vi "Autonomous Independent.vi"() -> ()   [LabVIEW 2018]
doc: "This VI is called when autonomous begins, and will automatically be terminated when autonomous ends. You can carry out timed or sensor driven robot movement independently without needing to return to the caller."
uses:
  State Machines/autos.ctl
  <vilib>/Rock Robotics/WPI/DriverStation/WPI_DriverStationRobotMode2.ctl
  Robot Global Data.vi
  <vilib>/Rock Robotics/Network Tables/NT Read Number.vi
  <vilib>/Rock Robotics/WPI/Utilities/WPI_GetSetVariantRefNum.vi
  Support Code/Valkyrie1Buttons.vi
panel:
  in  "Range":cluster{"output high":dbl, "output low":dbl}={"output high"=0.7, "output low"=-0.6}
  in  "Gains":T1={"proportional gain (Kc)"=0.03, "integral time (Ti, min)"=0.01, "derivative time (Td, min)"=0.0}
  in  "Time to stop R":i32=1000
  in  "Distance fwd r":dbl=700.0 format="%#_13g"
  in  "Time to Wait r":dbl=100.0
  in  "Distance fwd 1":dbl=200.0 format="%#_13g"
  in  "Time to stop":i32=1000
  out "Finished?":bool
  in  "Time to Wait":dbl=100.0
  # "Ganhos PID"
  # "Cargo Ship"
  # "Rocket"
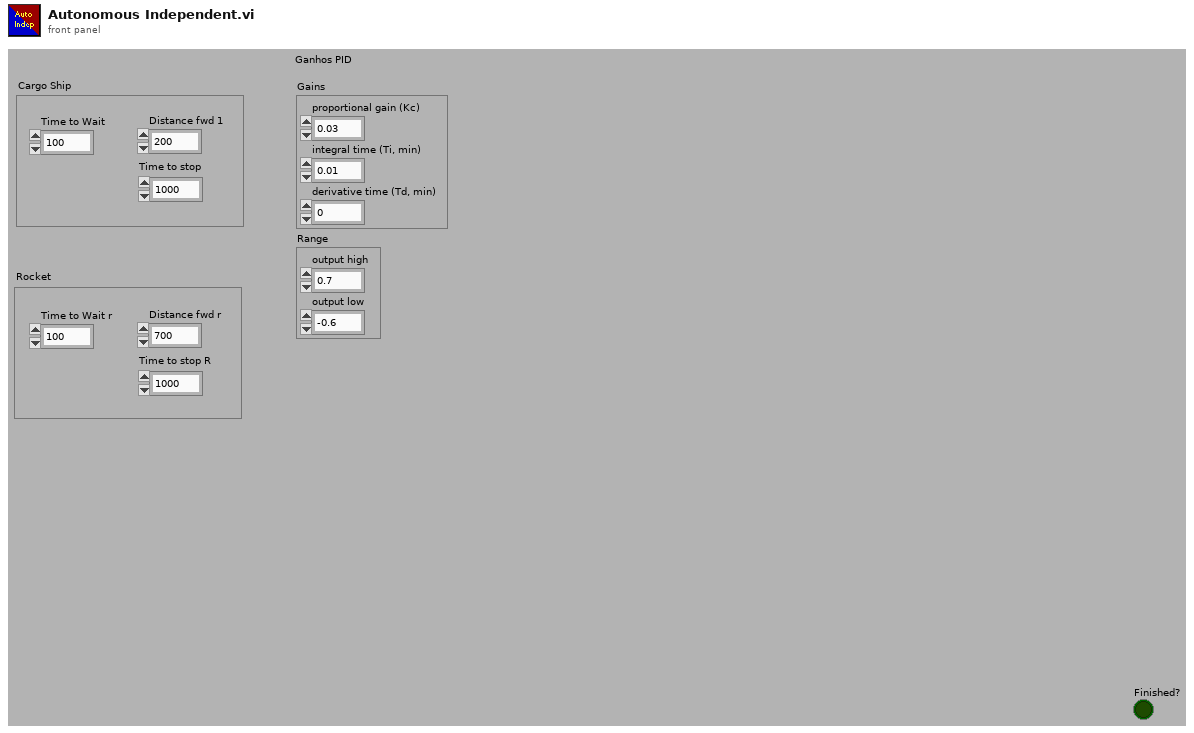
[diagram p1: front panel]
types:
  T1 = cluster{"proportional gain (Kc)":dbl, "integral time (Ti, min)":dbl, "derivative time (Td, min)":dbl}
  T2 = typedef "autos.ctl" = enum16{"Airship", " Rocket", "Anda"}
  T3 = enum16{"ZerandoSensor", "Frente1", "DriverAlinha", "Pontua", "Fim"}
  T4 = typedef "WPI_DriverStationRobotMode2.ctl" = enum16{"Autonomous Disabled", "Autonomous Enabled", "Teleop Disabled", "Teleop Enabled", "Disconnected", "Finish", "Test Disabled", "Test Enabled", "Emergency Stopped"}
  T5 = typedef "WPI_JoystickDevRef.ctl" = cluster{"Device":T6}
  T6 = typedef "WPI_JoystickDeviceEnum.ctl" = enum16{"USB 0", "USB 1", "USB 2", "USB 3", "USB 4", "USB 5"}
  T7 = typedef "D-Pad.ctl" = cluster{"Top":bool, "Bottom":bool, "None":bool, "Right":bool, "Left":bool}
  T8 = typedef "Button Cluster.ctl" = cluster{"Buttons[0]":bool, "Buttons[1]":bool, "Buttons[2]":bool, "Buttons[3]":bool, "Buttons[4]":bool, "Buttons[5]":bool, "Buttons[6]":bool, "Buttons[7]":bool, "Buttons[8]":bool, "Buttons[9]":bool}
  T9 = typedef "Axes Cluster.ctl" = cluster{"Axes[0]":dbl, "Axes[1]":dbl, "Axes[2]":dbl, "Axes[3]":dbl, "Axes[4]":dbl, "Axes[5]":dbl, "Axes[6]":dbl, "Axes[7]":dbl, "Axes[8]":dbl}
  T10 = typedef "WPI_EncoderDevRef.ctl" = cluster{"DevStatus":errorcluster, "EncoderIndex":T11, "CounterIndex":T12, "DistancePerCount":dbl, "Decoding Type":T13}
  T11 = typedef "FPGA_EncoderIdx.ctl" = enum8{"Enc 0", "Enc 1", "Enc 2", "Enc 3", "Enc 4", "Enc 5", "Enc 6", "Enc 7", "Invalid"}
  T12 = typedef "FPGA_CounterCtrSystemIndex.ctl" = enum8{"Ctr 0", "Ctr 1", "Ctr 2", "Ctr 3", "Ctr 4", "Ctr 5", "Ctr 6", "Ctr 7", "Invalid"}
  T13 = typedef "WPI_EncoderType.ctl" = enum16{"1x", "2x", "4x"}
  T14 = cluster{"Yaw":dbl, "Roll":dbl, "Pitch":dbl, "Heading":dbl, "Fused Heading":dbl}
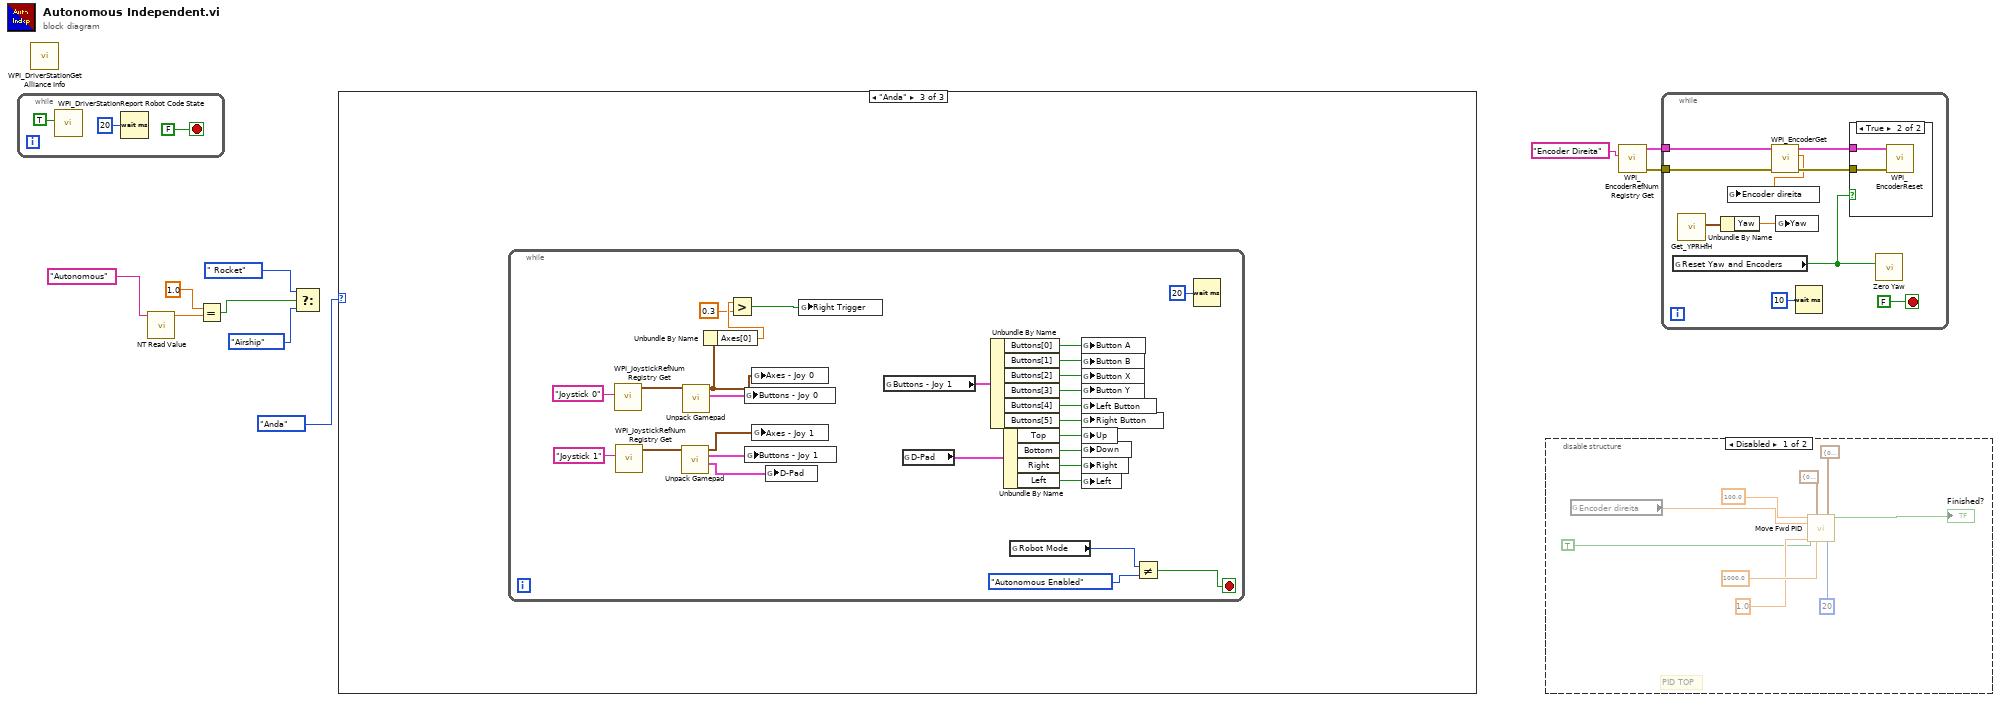
[diagram p0: block diagram]
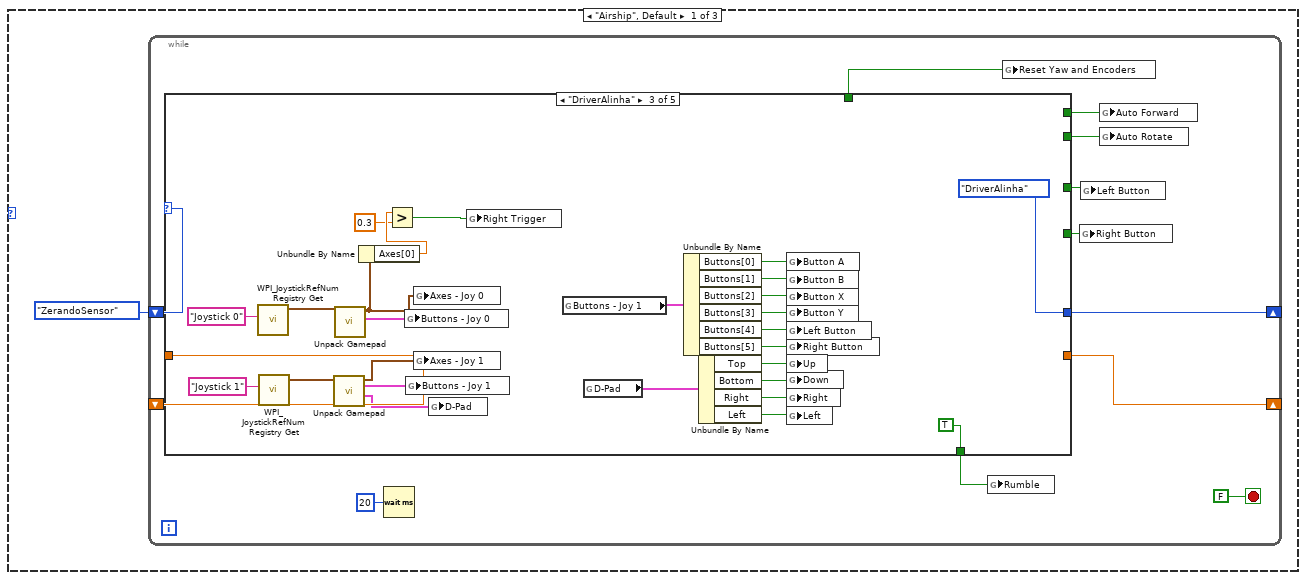
[diagram p4: hidden frame]
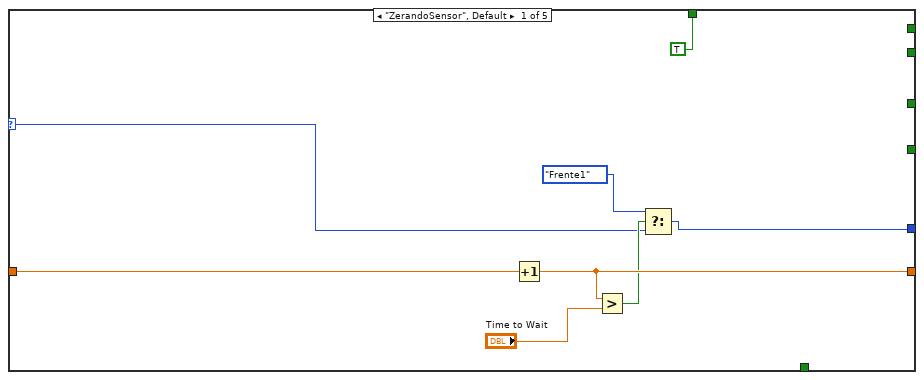
[diagram p5: hidden frame]
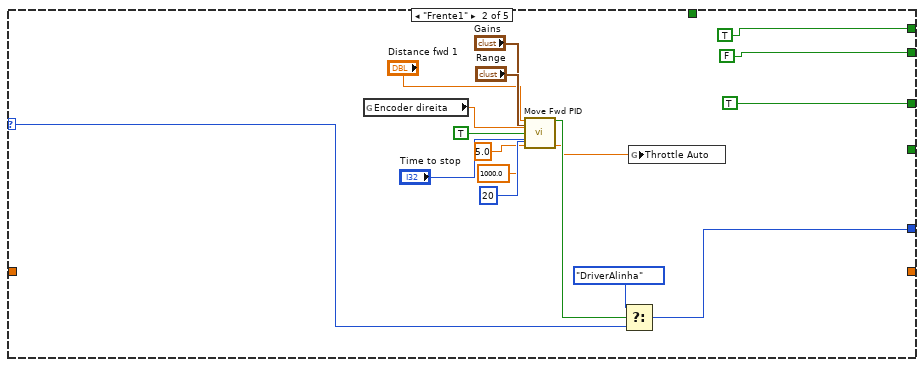
[diagram p6: hidden frame]
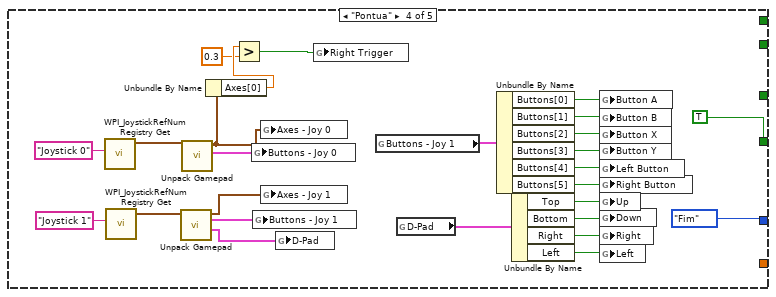
[diagram p7: hidden frame]
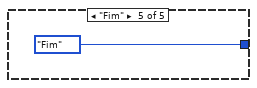
[diagram p8: hidden frame]
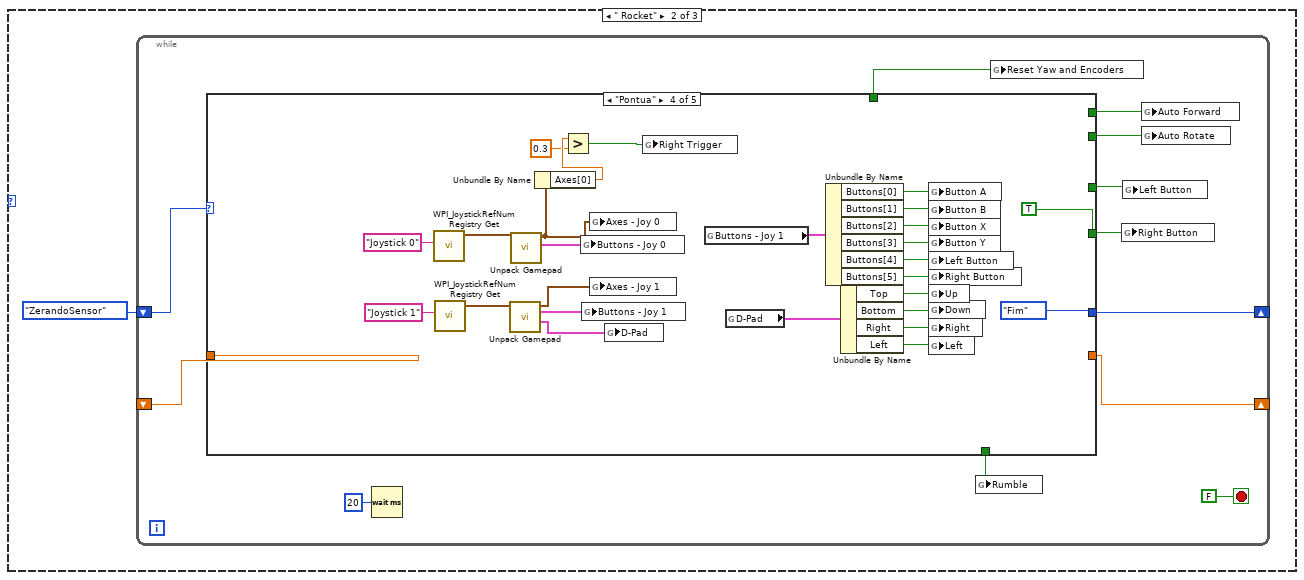
[diagram p9: hidden frame]
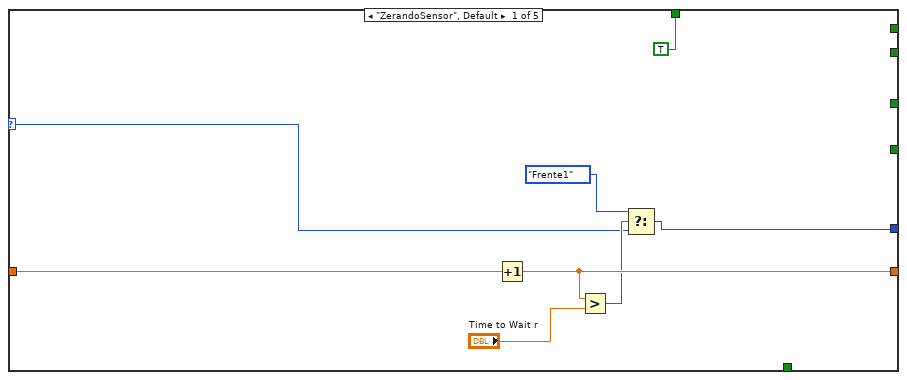
[diagram p10: hidden frame]
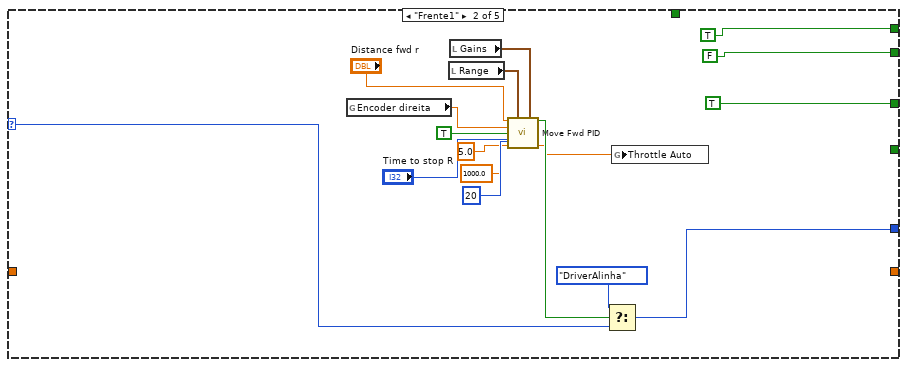
[diagram p11: hidden frame]
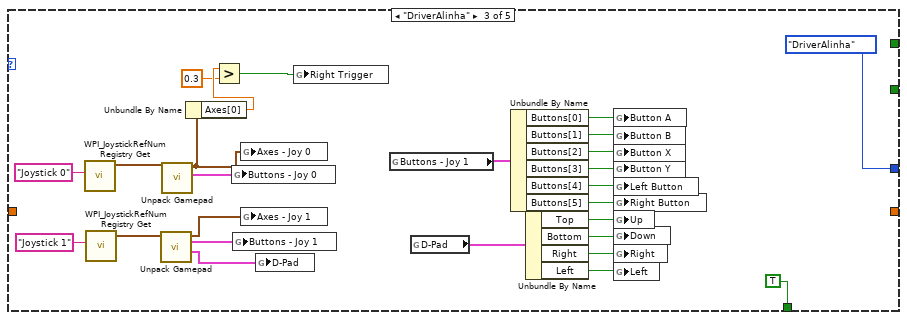
[diagram p12: hidden frame]
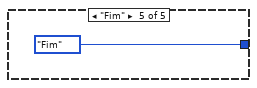
[diagram p13: hidden frame]
diagram:
  n1 = while {
    stop <- FALSE stop-if-true
    n2 = call <vilib>:"WPI_DriverStationReport Robot Code State.vi"("Autonomous"=TRUE) -> ()  [unwired: 10 in, 1 out]
    n3 = Wait (ms)(milliseconds to wait=u32 20) -> ()  [unwired: 1 out]
  }
  n4 = call <vilib>:"WPI_DriverStationGet Alliance Info.vi"() -> ()  [unwired: 12 out]
  n5 = call-poly <vilib>:"NT Read Value.vi"("Name"="Autonomous") -> ("Numeric"=w6:dbl)  [unwired: 9 in, 1 out]
  n6 = Equal?(x=1.0, y=w6) -> (x = y?=w2:bool)
  n7 = Select(t=autos." Rocket", s=w2, f=autos."Airship") -> ()  [unwired: 1 out]
  n8 = case shown="\"Anda\"" autos."Anda" {
    frame "Airship", Default {
      n9 = while {
        shift-right: [w23] -> _
        shift-left: _ -> [w24]
        shift-right: [w20] -> _
        shift-left: T3."ZerandoSensor" -> [w21]
        stop <- FALSE stop-if-true
        n10 = case shown="\"DriverAlinha\"" w21 {
          selector: w21 -> [w28 w50 _ _ _]
          tunnel: [TRUE _ _ _ _] -> w25
          tunnel: w24 -> [w33 _ _ _ _]
          tunnel: [w32 _ _ _ _] -> w23
          tunnel: [w30 w51 T3."DriverAlinha" ("t") T3."Fim" ("t") T3."Fim" ("t")] -> w20
          tunnel: [_ TRUE _ _ _] -> w19
          tunnel: [_ FALSE _ _ _] -> w18
          tunnel: [_ TRUE _ _ _] -> w17
          tunnel: [_ _ _ TRUE _] -> w16
          tunnel: [_ _ TRUE _ _] -> w15
          frame "ZerandoSensor", Default {
            n11 = Increment(x=w33) -> (x+1=w32:dbl)
            n12 = Greater?(x=w32, y="Time to Wait") -> (0:w29:bool)
            n13 = Select(t=T3."Frente1", s=w29, f=w28) -> (s? t:f=w30:T3)
          }
          frame "Frente1" {
            n14 = global read "Robot Global Data.vi" "Encoder direita"() -> (w48:dbl)
            n15 = call "Move Fwd PID.vi"("Distance"="Distance fwd 1", "Range"="Range", "Gains"="Gains", "Encoder Count"=w48, "Reset Rate"=TRUE, "Time to stop"="Time to stop", "Precision"=5.0, "Soft start"=1000.0, "Loop Timer"=20) -> ("Finished?"=w39:bool, "Output"=w35:dbl)  [unwired: 5 in]
            n16 = Select(t=T3."DriverAlinha", s=w39, f=w50) -> (s? t:f=w51:T3)
            n17 = global write "Robot Global Data.vi" "Throttle Auto"(w35) -> ()
          }
          frame "DriverAlinha" {
            n18 = call <vilib>:"WPI_JoystickRefNum Registry Get.vi"("refnum name"="Joystick 0") -> ("JoystickDevRef"=w74:T5)  [unwired: 1 in, 9 out]
            n19 = call <vilib>:"WPI_JoystickRefNum Registry Get.vi"("refnum name"="Joystick 1") -> ("JoystickDevRef"=w73:T5)  [unwired: 1 in, 9 out]
            n20 = call "Unpack Gamepad.vi"("JoystickDevRef"=w73) -> ("D-Pad"=w71:T7, "Button Cluster"=w70:T8, "Axes"=w69:T9)  [unwired: 8 in]
            n21 = call "Unpack Gamepad.vi"("JoystickDevRef"=w74) -> ("Button Cluster"=w72:T8, "Axes"=w68:T9)  [unwired: 8 in, 1 out]
            n22 = Unbundle By Name(w68) -> ("Axes[0]"=w67:dbl)
            n23 = Greater?(x=w67, y=0.3) -> (0:w65:bool)
            n24 = global write "Robot Global Data.vi" "Buttons - Joy 0"(w72) -> ()
            n25 = global write "Robot Global Data.vi" "Buttons - Joy 1"(w70) -> ()
            n26 = global write "Robot Global Data.vi" "Axes - Joy 0"(w68) -> ()
            n27 = global write "Robot Global Data.vi" "Axes - Joy 1"(w69) -> ()
            n28 = global write "Robot Global Data.vi" "D-Pad"(w71) -> ()
            n29 = global write "Valkyrie1Buttons.vi" "Right Trigger"(w65) -> ()
            n30 = global read "Robot Global Data.vi" "Buttons - Joy 1"() -> (w64:T8)
            n31 = global read "Robot Global Data.vi" "D-Pad"() -> (w63:T7)
            n32 = Unbundle By Name(w64) -> ("Buttons[0]"=w62:bool, "Buttons[1]"=w61:bool, "Buttons[2]"=w60:bool, "Buttons[3]"=w59:bool, "Buttons[4]"=w53:bool, "Buttons[5]"=w54:bool)
            n33 = Unbundle By Name(w63) -> ("Top"=w55:bool, "Bottom"=w56:bool, "Right"=w57:bool, "Left"=w58:bool)
            n34 = global write "Valkyrie1Buttons.vi" "Button A"(w62) -> ()
            n35 = global write "Valkyrie1Buttons.vi" "Button B"(w61) -> ()
            n36 = global write "Valkyrie1Buttons.vi" "Button X"(w60) -> ()
            n37 = global write "Valkyrie1Buttons.vi" "Button Y"(w59) -> ()
            n38 = global write "Valkyrie1Buttons.vi" "Left Button"(w53) -> ()
            n39 = global write "Valkyrie1Buttons.vi" "Right Button"(w54) -> ()
            n40 = global write "Valkyrie1Buttons.vi" "Up"(w55) -> ()
            n41 = global write "Valkyrie1Buttons.vi" "Down"(w56) -> ()
            n42 = global write "Valkyrie1Buttons.vi" "Right"(w57) -> ()
            n43 = global write "Valkyrie1Buttons.vi" "Left"(w58) -> ()
          }
          frame "Pontua" {
            n44 = call <vilib>:"WPI_JoystickRefNum Registry Get.vi"("refnum name"="Joystick 0") -> ("JoystickDevRef"=w99:T5)  [unwired: 1 in, 9 out]
            n45 = call <vilib>:"WPI_JoystickRefNum Registry Get.vi"("refnum name"="Joystick 1") -> ("JoystickDevRef"=w98:T5)  [unwired: 1 in, 9 out]
            n46 = call "Unpack Gamepad.vi"("JoystickDevRef"=w98) -> ("D-Pad"=w96:T7, "Button Cluster"=w95:T8, "Axes"=w94:T9)  [unwired: 8 in]
            n47 = call "Unpack Gamepad.vi"("JoystickDevRef"=w99) -> ("Button Cluster"=w97:T8, "Axes"=w81:T9)  [unwired: 8 in, 1 out]
            n48 = Unbundle By Name(w81) -> ("Axes[0]"=w80:dbl)
            n49 = Greater?(x=w80, y=0.3) -> (0:w78:bool)
            n50 = global write "Robot Global Data.vi" "Buttons - Joy 0"(w97) -> ()
            n51 = global write "Robot Global Data.vi" "Buttons - Joy 1"(w95) -> ()
            n52 = global write "Robot Global Data.vi" "Axes - Joy 0"(w81) -> ()
            n53 = global write "Robot Global Data.vi" "Axes - Joy 1"(w94) -> ()
            n54 = global write "Robot Global Data.vi" "D-Pad"(w96) -> ()
            n55 = global write "Valkyrie1Buttons.vi" "Right Trigger"(w78) -> ()
            n56 = global read "Robot Global Data.vi" "Buttons - Joy 1"() -> (w93:T8)
            n57 = global read "Robot Global Data.vi" "D-Pad"() -> (w92:T7)
            n58 = Unbundle By Name(w93) -> ("Buttons[0]"=w91:bool, "Buttons[1]"=w90:bool, "Buttons[2]"=w89:bool, "Buttons[3]"=w88:bool, "Buttons[4]"=w82:bool, "Buttons[5]"=w83:bool)
            n59 = Unbundle By Name(w92) -> ("Top"=w84:bool, "Bottom"=w85:bool, "Right"=w86:bool, "Left"=w87:bool)
            n60 = global write "Valkyrie1Buttons.vi" "Button A"(w91) -> ()
            n61 = global write "Valkyrie1Buttons.vi" "Button B"(w90) -> ()
            n62 = global write "Valkyrie1Buttons.vi" "Button X"(w89) -> ()
            n63 = global write "Valkyrie1Buttons.vi" "Button Y"(w88) -> ()
            n64 = global write "Valkyrie1Buttons.vi" "Left Button"(w82) -> ()
            n65 = global write "Valkyrie1Buttons.vi" "Right Button"(w83) -> ()
            n66 = global write "Valkyrie1Buttons.vi" "Up"(w84) -> ()
            n67 = global write "Valkyrie1Buttons.vi" "Down"(w85) -> ()
            n68 = global write "Valkyrie1Buttons.vi" "Right"(w86) -> ()
            n69 = global write "Valkyrie1Buttons.vi" "Left"(w87) -> ()
          }
          frame "Fim" {
          }
        }
        n70 = Wait (ms)(milliseconds to wait=u32 20) -> ()  [unwired: 1 out]
        n71 = global write "Robot Global Data.vi" "Rumble"(w15) -> ()
        n72 = global write "Robot Global Data.vi" "Reset Yaw and Encoders"(w25) -> ()
        n73 = global write "Valkyrie1Buttons.vi" "Right Button"(w16) -> ()
        n74 = global write "Valkyrie1Buttons.vi" "Left Button"(w17) -> ()
        n75 = global write "Robot Global Data.vi" "Auto Forward"(w19) -> ()
        n76 = global write "Robot Global Data.vi" "Auto Rotate"(w18) -> ()
      }
    }
    frame " Rocket" {
      n77 = while {
        shift-right: [w114] -> _
        shift-left: _ -> [w115]
        shift-right: [w111] -> _
        shift-left: T3."ZerandoSensor" -> [w112]
        stop <- FALSE stop-if-true
        n78 = case shown="\"Pontua\"" w112 {
          selector: w112 -> [w119 w141 _ _ _]
          tunnel: [TRUE _ _ _ _] -> w116
          tunnel: w115 -> [w124 _ _ _ _]
          tunnel: [w123 _ _ _ _] -> w114
          tunnel: [w121 w142 T3."DriverAlinha" ("t") T3."Fim" ("t") T3."Fim" ("t")] -> w111
          tunnel: [_ TRUE _ _ _] -> w110
          tunnel: [_ FALSE _ _ _] -> w109
          tunnel: [_ TRUE _ _ _] -> w108
          tunnel: [_ _ _ TRUE _] -> w107
          tunnel: [_ _ TRUE _ _] -> w106
          frame "ZerandoSensor", Default {
            n79 = Increment(x=w124) -> (x+1=w123:dbl)
            n80 = Greater?(x=w123, y="Time to Wait r") -> (0:w120:bool)
            n81 = Select(t=T3."Frente1", s=w120, f=w119) -> (s? t:f=w121:T3)
          }
          frame "Frente1" {
            n82 = global read "Robot Global Data.vi" "Encoder direita"() -> (w139:dbl)
            n83 = local read "Range"() -> (w126:cluster{"output high":dbl, "output low":dbl})
            n84 = local read "Gains"() -> (w127:T1)
            n85 = call "Move Fwd PID.vi"("Distance"="Distance fwd r", "Range"=w126, "Gains"=w127, "Encoder Count"=w139, "Reset Rate"=TRUE, "Time to stop"="Time to stop R", "Precision"=5.0, "Soft start"=1000.0, "Loop Timer"=20) -> ("Finished?"=w132:bool, "Output"=w128:dbl)  [unwired: 5 in]
            n86 = Select(t=T3."DriverAlinha", s=w132, f=w141) -> (s? t:f=w142:T3)
            n87 = global write "Robot Global Data.vi" "Throttle Auto"(w128) -> ()
          }
          frame "DriverAlinha" {
            n88 = call <vilib>:"WPI_JoystickRefNum Registry Get.vi"("refnum name"="Joystick 0") -> ("JoystickDevRef"=w165:T5)  [unwired: 1 in, 9 out]
            n89 = call <vilib>:"WPI_JoystickRefNum Registry Get.vi"("refnum name"="Joystick 1") -> ("JoystickDevRef"=w164:T5)  [unwired: 1 in, 9 out]
            n90 = call "Unpack Gamepad.vi"("JoystickDevRef"=w164) -> ("D-Pad"=w162:T7, "Button Cluster"=w161:T8, "Axes"=w160:T9)  [unwired: 8 in]
            n91 = call "Unpack Gamepad.vi"("JoystickDevRef"=w165) -> ("Button Cluster"=w163:T8, "Axes"=w159:T9)  [unwired: 8 in, 1 out]
            n92 = Unbundle By Name(w159) -> ("Axes[0]"=w158:dbl)
            n93 = Greater?(x=w158, y=0.3) -> (0:w156:bool)
            n94 = global write "Robot Global Data.vi" "Buttons - Joy 0"(w163) -> ()
            n95 = global write "Robot Global Data.vi" "Buttons - Joy 1"(w161) -> ()
            n96 = global write "Robot Global Data.vi" "Axes - Joy 0"(w159) -> ()
            n97 = global write "Robot Global Data.vi" "Axes - Joy 1"(w160) -> ()
            n98 = global write "Robot Global Data.vi" "D-Pad"(w162) -> ()
            n99 = global write "Valkyrie1Buttons.vi" "Right Trigger"(w156) -> ()
            n100 = global read "Robot Global Data.vi" "Buttons - Joy 1"() -> (w155:T8)
            n101 = global read "Robot Global Data.vi" "D-Pad"() -> (w154:T7)
            n102 = Unbundle By Name(w155) -> ("Buttons[0]"=w153:bool, "Buttons[1]"=w152:bool, "Buttons[2]"=w151:bool, "Buttons[3]"=w150:bool, "Buttons[4]"=w144:bool, "Buttons[5]"=w145:bool)
            n103 = Unbundle By Name(w154) -> ("Top"=w146:bool, "Bottom"=w147:bool, "Right"=w148:bool, "Left"=w149:bool)
            n104 = global write "Valkyrie1Buttons.vi" "Button A"(w153) -> ()
            n105 = global write "Valkyrie1Buttons.vi" "Button B"(w152) -> ()
            n106 = global write "Valkyrie1Buttons.vi" "Button X"(w151) -> ()
            n107 = global write "Valkyrie1Buttons.vi" "Button Y"(w150) -> ()
            n108 = global write "Valkyrie1Buttons.vi" "Left Button"(w144) -> ()
            n109 = global write "Valkyrie1Buttons.vi" "Right Button"(w145) -> ()
            n110 = global write "Valkyrie1Buttons.vi" "Up"(w146) -> ()
            n111 = global write "Valkyrie1Buttons.vi" "Down"(w147) -> ()
            n112 = global write "Valkyrie1Buttons.vi" "Right"(w148) -> ()
            n113 = global write "Valkyrie1Buttons.vi" "Left"(w149) -> ()
          }
          frame "Pontua" {
            n114 = call <vilib>:"WPI_JoystickRefNum Registry Get.vi"("refnum name"="Joystick 0") -> ("JoystickDevRef"=w190:T5)  [unwired: 1 in, 9 out]
            n115 = call <vilib>:"WPI_JoystickRefNum Registry Get.vi"("refnum name"="Joystick 1") -> ("JoystickDevRef"=w189:T5)  [unwired: 1 in, 9 out]
            n116 = call "Unpack Gamepad.vi"("JoystickDevRef"=w189) -> ("D-Pad"=w187:T7, "Button Cluster"=w186:T8, "Axes"=w185:T9)  [unwired: 8 in]
            n117 = call "Unpack Gamepad.vi"("JoystickDevRef"=w190) -> ("Button Cluster"=w188:T8, "Axes"=w172:T9)  [unwired: 8 in, 1 out]
            n118 = Unbundle By Name(w172) -> ("Axes[0]"=w171:dbl)
            n119 = Greater?(x=w171, y=0.3) -> (0:w169:bool)
            n120 = global write "Robot Global Data.vi" "Buttons - Joy 0"(w188) -> ()
            n121 = global write "Robot Global Data.vi" "Buttons - Joy 1"(w186) -> ()
            n122 = global write "Robot Global Data.vi" "Axes - Joy 0"(w172) -> ()
            n123 = global write "Robot Global Data.vi" "Axes - Joy 1"(w185) -> ()
            n124 = global write "Robot Global Data.vi" "D-Pad"(w187) -> ()
            n125 = global write "Valkyrie1Buttons.vi" "Right Trigger"(w169) -> ()
            n126 = global read "Robot Global Data.vi" "Buttons - Joy 1"() -> (w184:T8)
            n127 = global read "Robot Global Data.vi" "D-Pad"() -> (w183:T7)
            n128 = Unbundle By Name(w184) -> ("Buttons[0]"=w182:bool, "Buttons[1]"=w181:bool, "Buttons[2]"=w180:bool, "Buttons[3]"=w179:bool, "Buttons[4]"=w173:bool, "Buttons[5]"=w174:bool)
            n129 = Unbundle By Name(w183) -> ("Top"=w175:bool, "Bottom"=w176:bool, "Right"=w177:bool, "Left"=w178:bool)
            n130 = global write "Valkyrie1Buttons.vi" "Button A"(w182) -> ()
            n131 = global write "Valkyrie1Buttons.vi" "Button B"(w181) -> ()
            n132 = global write "Valkyrie1Buttons.vi" "Button X"(w180) -> ()
            n133 = global write "Valkyrie1Buttons.vi" "Button Y"(w179) -> ()
            n134 = global write "Valkyrie1Buttons.vi" "Left Button"(w173) -> ()
            n135 = global write "Valkyrie1Buttons.vi" "Right Button"(w174) -> ()
            n136 = global write "Valkyrie1Buttons.vi" "Up"(w175) -> ()
            n137 = global write "Valkyrie1Buttons.vi" "Down"(w176) -> ()
            n138 = global write "Valkyrie1Buttons.vi" "Right"(w177) -> ()
            n139 = global write "Valkyrie1Buttons.vi" "Left"(w178) -> ()
          }
          frame "Fim" {
          }
        }
        n140 = Wait (ms)(milliseconds to wait=u32 20) -> ()  [unwired: 1 out]
        n141 = global write "Robot Global Data.vi" "Rumble"(w106) -> ()
        n142 = global write "Robot Global Data.vi" "Reset Yaw and Encoders"(w116) -> ()
        n143 = global write "Valkyrie1Buttons.vi" "Right Button"(w107) -> ()
        n144 = global write "Valkyrie1Buttons.vi" "Left Button"(w108) -> ()
        n145 = global write "Robot Global Data.vi" "Auto Forward"(w110) -> ()
        n146 = global write "Robot Global Data.vi" "Auto Rotate"(w109) -> ()
      }
    }
    frame "Anda" {
      n147 = while {
        stop <- w196 stop-if-true
        n148 = call <vilib>:"WPI_JoystickRefNum Registry Get.vi"("refnum name"="Joystick 0") -> ("JoystickDevRef"=w221:T5)  [unwired: 1 in, 9 out]
        n149 = call <vilib>:"WPI_JoystickRefNum Registry Get.vi"("refnum name"="Joystick 1") -> ("JoystickDevRef"=w220:T5)  [unwired: 1 in, 9 out]
        n150 = call "Unpack Gamepad.vi"("JoystickDevRef"=w220) -> ("D-Pad"=w218:T7, "Button Cluster"=w217:T8, "Axes"=w216:T9)  [unwired: 8 in]
        n151 = call "Unpack Gamepad.vi"("JoystickDevRef"=w221) -> ("Button Cluster"=w219:T8, "Axes"=w215:T9)  [unwired: 8 in, 1 out]
        n152 = Unbundle By Name(w215) -> ("Axes[0]"=w214:dbl)
        n153 = Greater?(x=w214, y=0.3) -> (0:w212:bool)
        n154 = global write "Robot Global Data.vi" "Buttons - Joy 0"(w219) -> ()
        n155 = global write "Robot Global Data.vi" "Buttons - Joy 1"(w217) -> ()
        n156 = global write "Robot Global Data.vi" "Axes - Joy 0"(w215) -> ()
        n157 = global write "Robot Global Data.vi" "Axes - Joy 1"(w216) -> ()
        n158 = global write "Robot Global Data.vi" "D-Pad"(w218) -> ()
        n159 = global write "Valkyrie1Buttons.vi" "Right Trigger"(w212) -> ()
        n160 = global read "Robot Global Data.vi" "Buttons - Joy 1"() -> (w211:T8)
        n161 = global read "Robot Global Data.vi" "D-Pad"() -> (w210:T7)
        n162 = Unbundle By Name(w211) -> ("Buttons[0]"=w209:bool, "Buttons[1]"=w208:bool, "Buttons[2]"=w207:bool, "Buttons[3]"=w206:bool, "Buttons[4]"=w200:bool, "Buttons[5]"=w201:bool)
        n163 = Unbundle By Name(w210) -> ("Top"=w202:bool, "Bottom"=w203:bool, "Right"=w204:bool, "Left"=w205:bool)
        n164 = global read "Robot Global Data.vi" "Robot Mode"() -> (w198:T4)
        n165 = global write "Valkyrie1Buttons.vi" "Button A"(w209) -> ()
        n166 = global write "Valkyrie1Buttons.vi" "Button B"(w208) -> ()
        n167 = global write "Valkyrie1Buttons.vi" "Button X"(w207) -> ()
        n168 = global write "Valkyrie1Buttons.vi" "Button Y"(w206) -> ()
        n169 = global write "Valkyrie1Buttons.vi" "Left Button"(w200) -> ()
        n170 = global write "Valkyrie1Buttons.vi" "Right Button"(w201) -> ()
        n171 = global write "Valkyrie1Buttons.vi" "Up"(w202) -> ()
        n172 = global write "Valkyrie1Buttons.vi" "Down"(w203) -> ()
        n173 = global write "Valkyrie1Buttons.vi" "Right"(w204) -> ()
        n174 = global write "Valkyrie1Buttons.vi" "Left"(w205) -> ()
        n175 = Not Equal?(x=w198, y=WPI_DriverStationRobotMode2."Autonomous Enabled" ("x")) -> (x != y?=w196:bool)
        n176 = Wait (ms)(milliseconds to wait=u32 20) -> ()  [unwired: 1 out]
      }
    }
  }
  n177 = disable-structure shown="Disabled" {
    frame Disabled {
      # "PID TOP"
      n178 = global read "Robot Global Data.vi" "Encoder direita"() -> (w232:dbl)
      n179 = call "Move Fwd PID.vi"("Distance"=100.0, "Range"=cluster{"output high":dbl, "output low":dbl} {"output high"=0.7, "output low"=-0.6}, "Gains"=T1 {"proportional gain (Kc)"=0.03, "integral time (Ti, min)"=0.01, "derivative time (Td, min)"=0.0}, "Encoder Count"=w232, "Reset Rate"=TRUE, "Precision"=1.0, "Soft start"=1000.0, "Loop Timer"=20) -> ("Finished?"=→"Finished?":bool)  [unwired: 6 in, 1 out]
    }
    frame Enabled {
    }
  }
  n180 = call <vilib>:"WPI_EncoderRefNum Registry Get.vi"("refnum name"="Encoder Direita") -> ("error out"=w8:errorcluster, "EncoderDevRef"=w9:T10)  [unwired: 9 in]
  n181 = while {
    tunnel: w9 -> [w241]
    tunnel: w8 -> [w240]
    stop <- FALSE stop-if-true
    n182 = global read "Robot Global Data.vi" "Reset Yaw and Encoders"() -> (w236:bool)
    n183 = call <vilib>:"Get_YPRHfH.vi"() -> ("YRPHfH"=w239:T14)  [unwired: 11 in]
    n184 = Unbundle By Name(w239) -> ("Yaw"=w233:dbl)
    n185 = call <vilib>:"WPI_EncoderGet.vi"("error in (no error)"=w240, "EncoderDevRef"=w241) -> ("error out"=w237:errorcluster, "Distance"=w234:dbl, "EncoderDevRef"=w238:T10)  [unwired: 4 in, 3 out]
    n186 = global write "Robot Global Data.vi" "Encoder direita"(w234) -> ()
    n187 = global write "Robot Global Data.vi" "Yaw"(w233) -> ()
    n188 = Wait (ms)(milliseconds to wait=u32 10) -> ()  [unwired: 1 out]
    n189 = case shown="True" w236 {
      tunnel: w238 -> [_ w244]
      tunnel: w237 -> [_ w243]
      frame False {
      }
      frame True {
        n190 = call <vilib>:"WPI_EncoderReset.vi"("error in (no error)"=w243, "EncoderDevRef"=w244) -> ()  [unwired: 8 in, 2 out]
      }
    }
    n191 = call <vilib>:"Zero Yaw.vi"("Zero"=w236) -> ()  [unwired: 11 in]
  }
